vi "Get Plot ID.vi"(8 "error in (no error)":errorcluster, 11 "3D Bar Datatype.lvclass in":refnum<class "3D Bar Datatype.lvclass">) -> (0 "error out":errorcluster, 1 "Plot ID":i32, 3 "3D Bar Datatype.lvclass out":refnum<class "3D Bar Datatype.lvclass">)   [LabVIEW 2017, in "3D Bar Datatype.lvclass"]
uses:
  <vilib>/Math Plots/3D Math Plots/3D Bar/3D Bar Datatype/3D Bar Datatype.lvclass
  <vilib>/Math Plots/3D Math Plots/3D Bar/3D Bar Datatype/3D Bar Datatype.lvclass/3D Bar Datatype.ctl
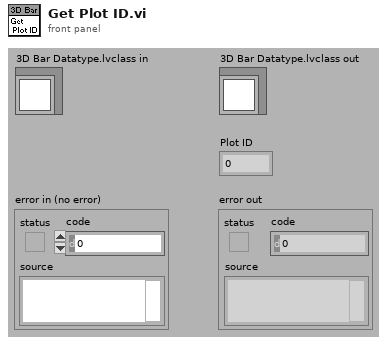
[diagram p1: front panel]
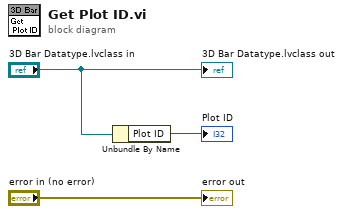
[diagram p0: block diagram]
diagram:
  n1 = Unbundle By Name("3D Bar Datatype.lvclass in") -> ("Plot ID"=→"Plot ID":i32)
  "3D Bar Datatype.lvclass out" <- "3D Bar Datatype.lvclass in"
  "error out" <- "error in (no error)"
